vi "Project.vi"(0 "I":dbl=1e-06 min=1e-09 max=1.0 step=1e-06 format="%.4e", 1 "Ti":dbl min=0.0 max=400.0 format="%.3f", 7 "Measurement":bool=TRUE, 8 "Auto\nTemp?":bool=TRUE) -> ()   [LabVIEW 2012]
uses:
  subVIs/Control 1.ctl
panel:
  in  "Tf":dbl=4.0 min=0.0 max=400.0 format="%.3f"
  out "?":cluster{"X":dbl, "Y":dbl}[](graph)
  out "?":cluster{dbl, dbl}[](graph)
  in  "Volt Delay 2":u32=50
  out "R/Ohm 2":dbl=1e-09 min=-1.0 step=1e-09 format="%.3e"
  out "T/K 2":dbl min=0.0 step=0.01 format="%.3f"
  in  "Ramp":ext format="%.3f"
  in  "Range":dbl=3.0 format="%.2f"
  in  "Y data precision":T1=7.0
  in  "X data precision":T1=3.0
  in  "Path":path
  in  "File name":string
  in  "Autorange":bool=TRUE
  in  "Voltmeter PLC":dbl=1.0 min=0.01 max=60.0 step=0.01 format="%.2f"
  in  "Voltage Compliance":dbl=12.0 min=0.1 max=105.0 step=0.1 format="%.2f"
  in  "minutes to wait before start":u32=5
  in  "Delay time":sgl min=0 step=1 format="%.2f"
  # "ON"
  # "OFF"
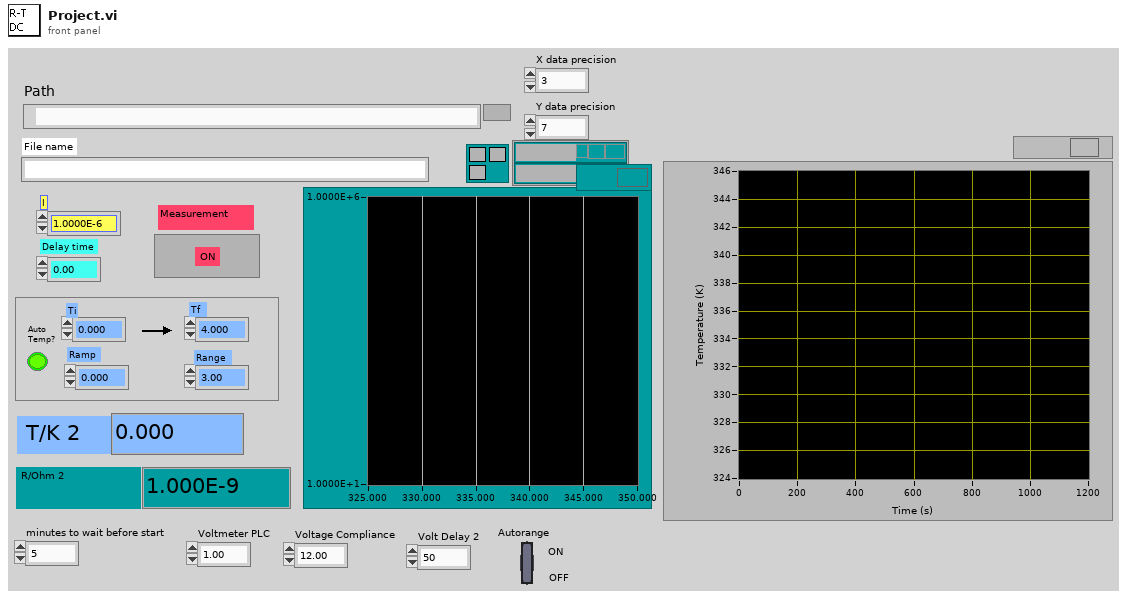
[diagram p1: front panel]
types:
  T1 = typedef "Control 1.ctl" = dbl
  T2 = enum16{"open", "replace", "create", "open or create", "replace or create", "replace or create with confirmation"}
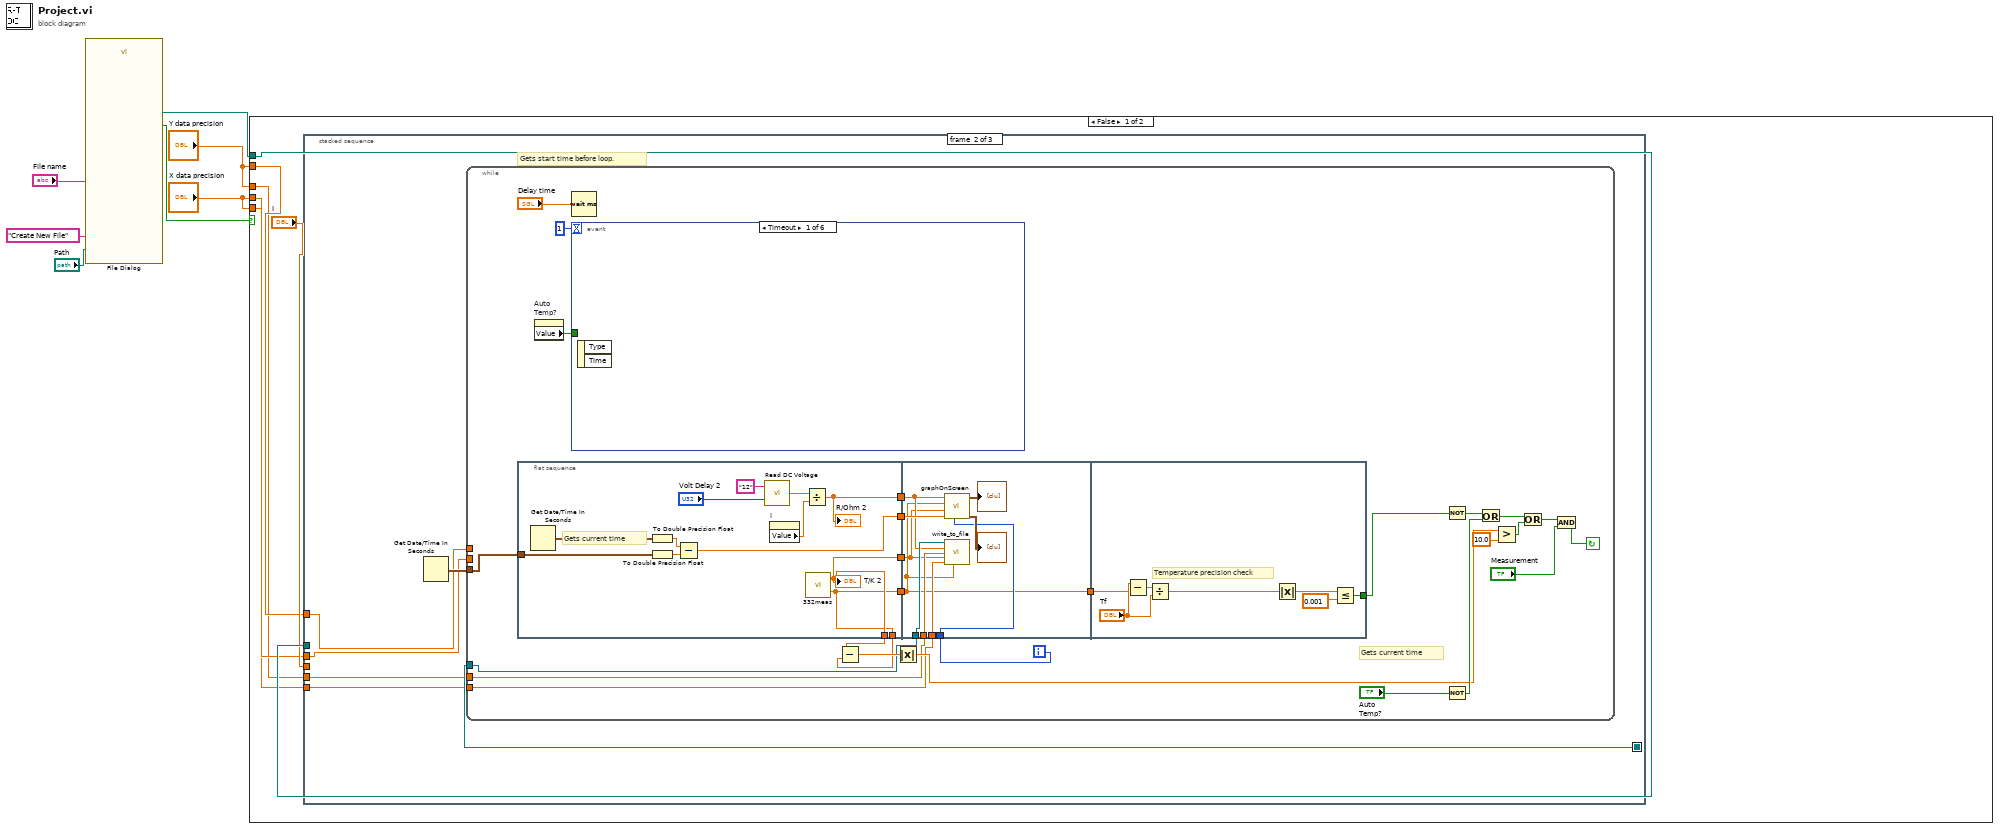
[diagram p0: block diagram]
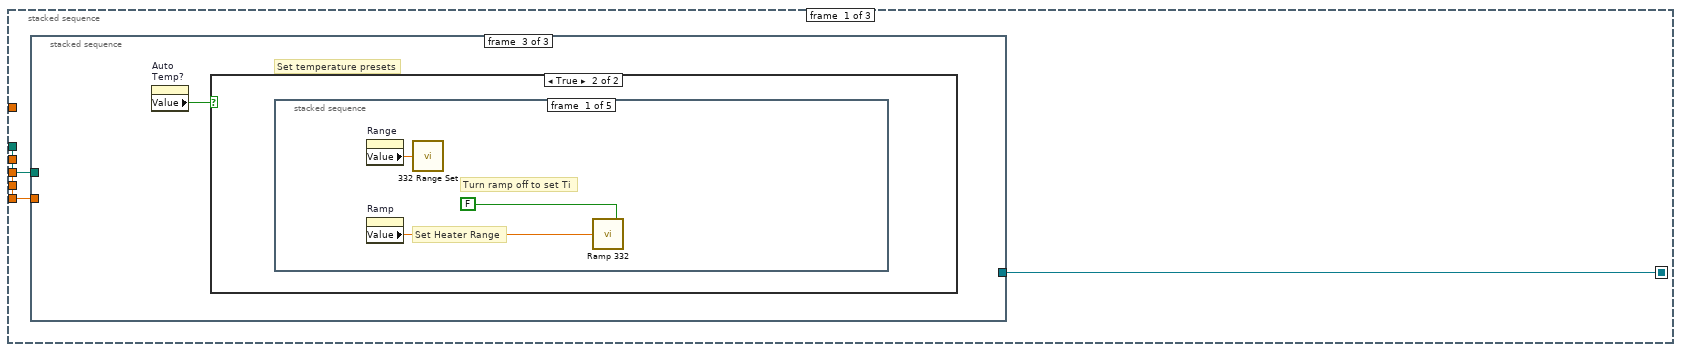
[diagram p2: hidden frame]
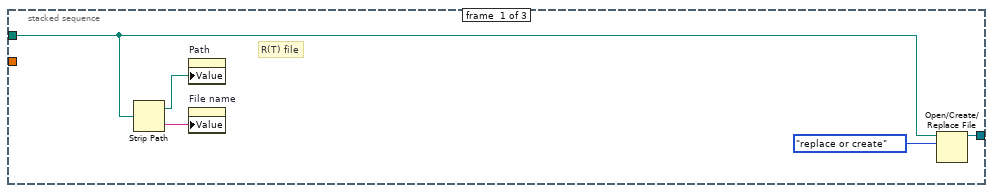
[diagram p3: hidden frame]
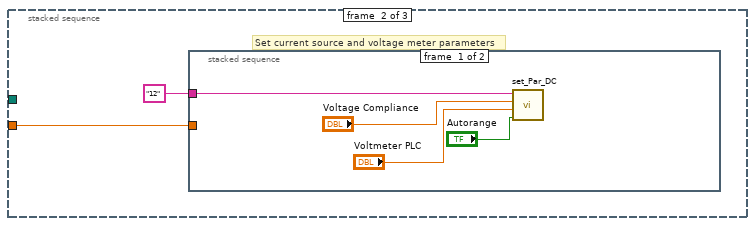
[diagram p4: hidden frame]
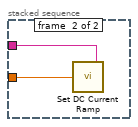
[diagram p5: hidden frame]
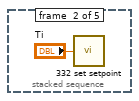
[diagram p7: hidden frame]
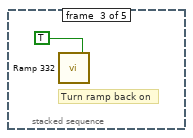
[diagram p8: hidden frame]
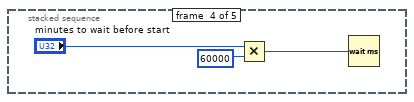
[diagram p9: hidden frame]
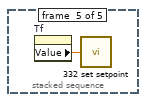
[diagram p10: hidden frame]
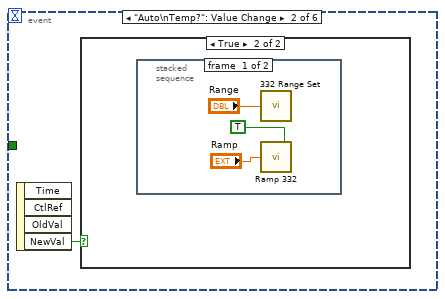
[diagram p11: hidden frame]
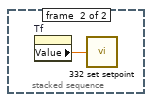
[diagram p13: hidden frame]
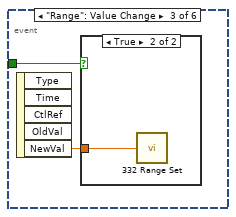
[diagram p14: hidden frame]
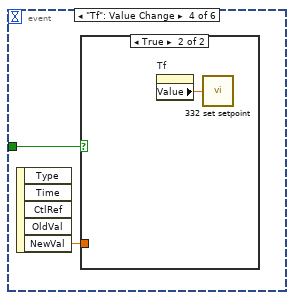
[diagram p16: hidden frame]
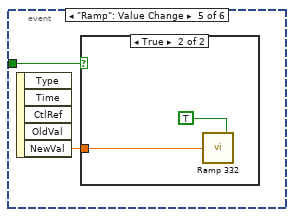
[diagram p18: hidden frame]
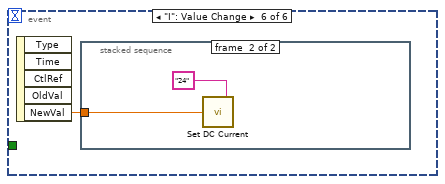
[diagram p20: hidden frame]
diagram:
  n1 = call "File Dialog"("start path"="Path", "prompt"="Create New File", "default name"="File name") -> ("selected path"=w4:path, "cancelled"=w3:bool)  [unwired: 9 in, 2 out]
  n2 = case shown="False" w3 {
    tunnel: w4 -> [w13 _]
    tunnel: "Y data precision" -> [w11 _]
    tunnel: "X data precision" -> [w10 _]
    tunnel: "Y data precision" -> [w9 _]
    tunnel: "X data precision" -> [w8 _]
    frame False {
      n3 = stacked-sequence {
        seq-local: [w16 _ _] -> [_ w42 w124]
        tunnel: "I" -> [w15 _ w121]
        tunnel: w13 -> [w14 _ _]
        tunnel: w11 -> [_ w44 _]
        tunnel: w10 -> [_ w43 _]
        tunnel: w9 -> [_ w41 _]
        tunnel: w8 -> [_ w40 _]
        frame #0 {
          n4 = stacked-sequence {
            tunnel: [w21 _ _] -> w16
            tunnel: w15 -> [_ w22 _]
            tunnel: w14 -> [w17 _ _]
            frame #0 {
              # "R(T) file"
              n5 = Strip Path(path=w17) -> (stripped path=w18:path, name=w19:string)
              n6 = property on="Path" class="Path"("Value"=w18) -> ()  [unwired: 2 in, 2 out]
              n7 = property on="File name" class="Str"("Value"=w19) -> ()  [unwired: 2 in, 2 out]
              n8 = Open/Create/Replace File(file path (use dialog)=w17, operation (0:open)=T2."replace or create") -> (refnum out=w21:refnum<file>)  [unwired: 4 in, 2 out]
            }
            frame #1 {
              # "Set current source and voltage meter parameters"
              n9 = stacked-sequence {
                tunnel: "12" ("Address") -> [w27 w29]
                tunnel: w22 -> [_ w28]
                frame #0 {
                  n10 = call "set_Par_DC.vi"("Autorange"="Autorange", "Voltmeter PLC"="Voltmeter PLC", "Voltage Compliance"="Voltage Compliance", "Address"=w27) -> ()
                }
                frame #1 {
                  n11 = call "Set DC Current Ramp.vi"("Address"=w29, "Current"=w28) -> ()
                }
              }
            }
            frame #2 {
              # "Set temperature presets"
              n12 = property on="Auto\nTemp?" class="Bool (strict)"() -> ("Value"=w30:bool)  [unwired: 2 in, 2 out]
              n13 = case shown="True" w30 {
                frame False {
                }
                frame True {
                  n14 = stacked-sequence {
                    frame #0 {
                      # "Set Heater Range"
                      # "Turn ramp off to set Ti"
                      n15 = property on="Range" class="DigNum (strict)"() -> ("Value"=w32:dbl)  [unwired: 2 in, 2 out]
                      n16 = property on="Ramp" class="DigNum (strict)"() -> ("Value"=w31:ext)  [unwired: 2 in, 2 out]
                      n17 = call "332 Range Set.vi"("Power Range: 93C\n0=OFF, 1=Low, 2=Med, 3=High"=w32) -> ()
                      n18 = call "Ramp 332.vi"("On"=FALSE, "K/min"=w31) -> ()
                    }
                    frame #1 {
                      n19 = call "332 set setpoint.vi"("Set Temperature SetPoint:332"="Ti") -> ()
                    }
                    frame #2 {
                      # "Turn ramp back on"
                      n20 = call "Ramp 332.vi"("On"=TRUE) -> ()  [unwired: 1 in]
                    }
                    frame #3 {
                      n21 = Multiply(x="minutes to wait before start", y=u32 60000) -> (x*y=w37:u32)
                      n22 = Wait (ms)(milliseconds to wait=w37) -> ()  [unwired: 1 out]
                    }
                    frame #4 {
                      n23 = property on="Tf" class="DigNum (strict)"() -> ("Value"=w39:dbl)  [unwired: 2 in, 2 out]
                      n24 = call "332 set setpoint.vi"("Set Temperature SetPoint:332"=w39) -> ()
                    }
                  }
                }
              }
            }
          }
        }
        frame #1 {
          # "Gets start time before loop."
          n25 = Get Date/Time In Seconds() -> (seconds since 1Jan1904=w45:timestamp)
          n26 = while {
            tunnel: w45 -> [w53]
            tunnel: w44 -> [_]
            tunnel: w43 -> [_]
            tunnel: w42 -> [w60]
            tunnel: w41 -> [w55]
            tunnel: w40 -> [w54]
            i -> [w56]
            stop <- w72 continue-if-true
            # "Gets current time"
            n27 = flat-sequence {
              tunnel: [w95] -> w59
              tunnel: [w96] -> w58
              tunnel: [w93] -> w57
              tunnel: w53 -> [w94]
              tunnel: [w93] -> w52
              tunnel: [w92] -> w51
              tunnel: [w92] -> w49
              tunnel: w60 -> [w111]
              tunnel: w59 -> [w106]
              tunnel: w58 -> [w110]
              tunnel: w57 -> [w104]
              tunnel: w56 -> [w109]
              tunnel: w55 -> [w108]
              tunnel: w54 -> [w107]
              tunnel: w49 -> [w105]
              tunnel: [w105] -> w48
              tunnel: [w115] -> w50
              tunnel: w48 -> [w114]
              frame #0 {
                # "Gets current time"
                n28 = Get Date/Time In Seconds() -> (seconds since 1Jan1904=w98:timestamp)
                n29 = To Double Precision Float(number=w98) -> (double precision float=w99:dbl)
                n30 = To Double Precision Float(number=w94) -> (double precision float=w97:dbl)
                n31 = Subtract(x=w99, y=w97) -> (x-y=w96:dbl)
                n32 = call "Read DC Voltage.vi"("Volt Delay"="Volt Delay 2", "Address"="12" ("address string")) -> ("Voltage"=w101:dbl)
                n33 = property on="I" class="DigNum (strict)"() -> ("Value"=w102:dbl)  [unwired: 2 in, 2 out]
                n34 = Divide(x=w101, y=w102) -> (x/y=w95:dbl)
                "R/Ohm 2" <- w95
                n35 = call "332meas.vi"() -> ("332 Temp [K]"=w93:dbl, "332 Temp Setpoint [K]"=w92:dbl)  [unwired: 1 in]
                "T/K 2" <- w93
              }
              frame #1 {
                n36 = call "graphOnScreen.vi"("Connect to loop iteration"=w109, "Time"=w110, "332 Temp [K]"=w104, "332 Temp Setpoint [K]"=w105, "R(ohm)"=w106) -> ("T(t)"=→"?":cluster{"X":dbl, "Y":dbl}[], 3:→"?":cluster{dbl, dbl}[])  [unwired: 5 in]
                n37 = call "write_to_file.vi"("refnum"=w111, "y data"=w106, "y data precision"=w108, "x data"=w104, "x data precision"=w107, "Setpoint"=w105) -> ()  [unwired: 10 in]
              }
              frame #2 {
                # "Temperature precision check"
                n38 = Subtract(x="Tf", y=w114) -> (x-y=w118:dbl)
                n39 = Divide(x=w118, y="Tf") -> (x/y=w119:dbl)
                n40 = Absolute Value(x=w119) -> (abs(x)=w117:dbl)
                n41 = Less Or Equal?(x=w117, y=0.001) -> (x <= y?=w115:bool)
              }
            }
            n42 = property on="Auto\nTemp?" class="Bool (strict)"() -> ("Value"=w47:bool)  [unwired: 2 in, 2 out]
            n43 = Wait (ms)(milliseconds to wait="Delay time") -> ()  [unwired: 1 out]
            n44 = event shown="[0] Timeout" {
              selector: _ -> [_ _ _ _ _ _]
              dyn-events: _ -> [_ _ _ _ _ _]
              timeout: 1 -> [_ _ _ _ _ _]
              tunnel: w47 -> [_ _ w78 w81 w84 _]
              event Timeout {
                n45 = event-data() -> ()  [unwired: 1 in, 2 out]
              }
              event "Auto\nTemp?": Value Change {
                n46 = event-data() -> ("NewVal"=w73:bool)  [unwired: 1 in, 3 out]
                n47 = case shown="True" w73 {
                  frame False {
                  }
                  frame True {
                    n48 = stacked-sequence {
                      frame #0 {
                        n49 = call "332 Range Set.vi"("Power Range: 93C\n0=OFF, 1=Low, 2=Med, 3=High"="Range") -> ()
                        n50 = call "Ramp 332.vi"("On"=TRUE, "K/min"="Ramp") -> ()
                      }
                      frame #1 {
                        n51 = property on="Tf" class="DigNum (strict)"() -> ("Value"=w77:dbl)  [unwired: 2 in, 2 out]
                        n52 = call "332 set setpoint.vi"("Set Temperature SetPoint:332"=w77) -> ()
                      }
                    }
                  }
                }
              }
              event "Range": Value Change {
                n53 = event-data() -> ("NewVal"=w79:dbl)  [unwired: 1 in, 4 out]
                n54 = case shown="True" w78 {
                  tunnel: w79 -> [_ w80]
                  frame False {
                  }
                  frame True {
                    n55 = call "332 Range Set.vi"("Power Range: 93C\n0=OFF, 1=Low, 2=Med, 3=High"=w80) -> ()
                  }
                }
              }
              event "Tf": Value Change {
                n56 = event-data() -> ("NewVal"=w82:dbl)  [unwired: 1 in, 4 out]
                n57 = case shown="True" w81 {
                  tunnel: w82 -> [_ _]
                  frame False {
                  }
                  frame True {
                    n58 = property on="Tf" class="DigNum (strict)"() -> ("Value"=w83:dbl)  [unwired: 2 in, 2 out]
                    n59 = call "332 set setpoint.vi"("Set Temperature SetPoint:332"=w83) -> ()
                  }
                }
              }
              event "Ramp": Value Change {
                n60 = event-data() -> ("NewVal"=w85:ext)  [unwired: 1 in, 4 out]
                n61 = case shown="True" w84 {
                  tunnel: w85 -> [_ w86]
                  frame False {
                  }
                  frame True {
                    n62 = call "Ramp 332.vi"("On"=TRUE, "K/min"=w86) -> ()
                  }
                }
              }
              event "I": Value Change {
                n63 = event-data() -> ("NewVal"=w88:dbl)  [unwired: 1 in, 4 out]
                n64 = stacked-sequence {
                  tunnel: w88 -> [_ w90]
                  frame #0 {
                    # "Wait until measurement\nfinished"
                    n65 = Wait (ms)(milliseconds to wait=u32 1000) -> ()  [unwired: 1 out]
                  }
                  frame #1 {
                    n66 = call "Set DC Current.vi"("Address"="24" ("address string"), "Current"=w90) -> ()
                  }
                }
              }
            }
            n67 = Subtract(x=w52, y=w51) -> (x-y=w66:dbl)
            n68 = Absolute Value(x=w66) -> (abs(x)=w62:dbl)
            n69 = Not(x=w50) -> (.not. x?=w70:bool)
            n70 = Not(x="Auto\nTemp?") -> (.not. x?=w67:bool)
            n71 = Or(x=w70, y=w67) -> (x .or. y?=w65:bool)
            n72 = Greater?(x=w62, y=10.0) -> (0:w61:bool)
            n73 = Or(x=w65, y=w61) -> (x .or. y?=w64:bool)
            n74 = And(x=w64, y="Measurement") -> (x .and. y?=w72:bool)
          }
        }
        frame #2 {
          w122 = "12" ("Address")
          n75 = call "Send to Volt Meter.vi"("Address"=w122, "Data"=":trig:sour imm;:init") -> ()
          n76 = stacked-sequence {
            tunnel: w122 -> [w126 w127]
            tunnel: w121 -> [w125 _]
            frame #0 {
              n77 = call "Set DC Current Ramp to Zero.vi"("Address"=w126, "Current"=w125) -> ()
            }
            frame #1 {
              n78 = call "disarm.vi"("address string"=w127) -> ()  [unwired: 1 in, 1 out]
            }
          }
          n79 = Close File(refnum=w124) -> ()  [unwired: 1 in, 2 out]
        }
      }
    }
    frame True {
    }
  }
